vi "Test.vi"(8 "error in (no error)":errorcluster, 10 "board image":T1, 11 "DAQ Board Design in":refnum<class "DAQ Board Design.lvclass">) -> (0 "error out":errorcluster, 2 "pass?":T2, 3 "Test name":string)   [LabVIEW 2018, in "DAQ Board Design.lvclass"]
doc: "Image check for blocks that are common to all types of boards."
uses:
  DAQ Board Design.lvclass
  Common/Pass Fail Boolean.ctl
  Common/Board Image.ctl
  Board Design_class/Board Design.lvclass
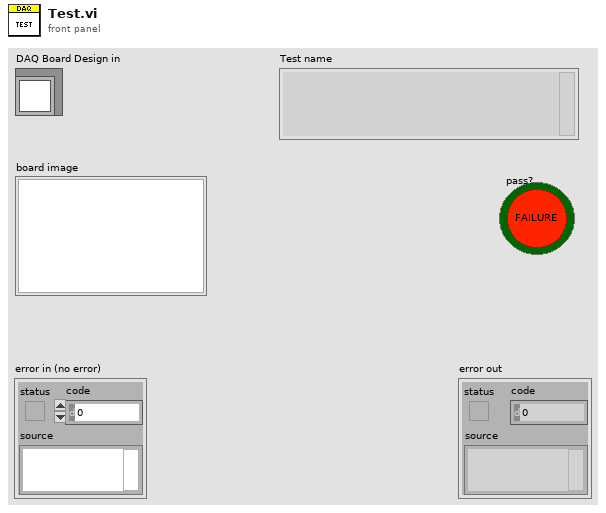
[diagram p1: front panel]
types:
  T1 = typedef "Board Image.ctl" = picture
  T2 = typedef "Pass Fail Boolean.ctl" = bool
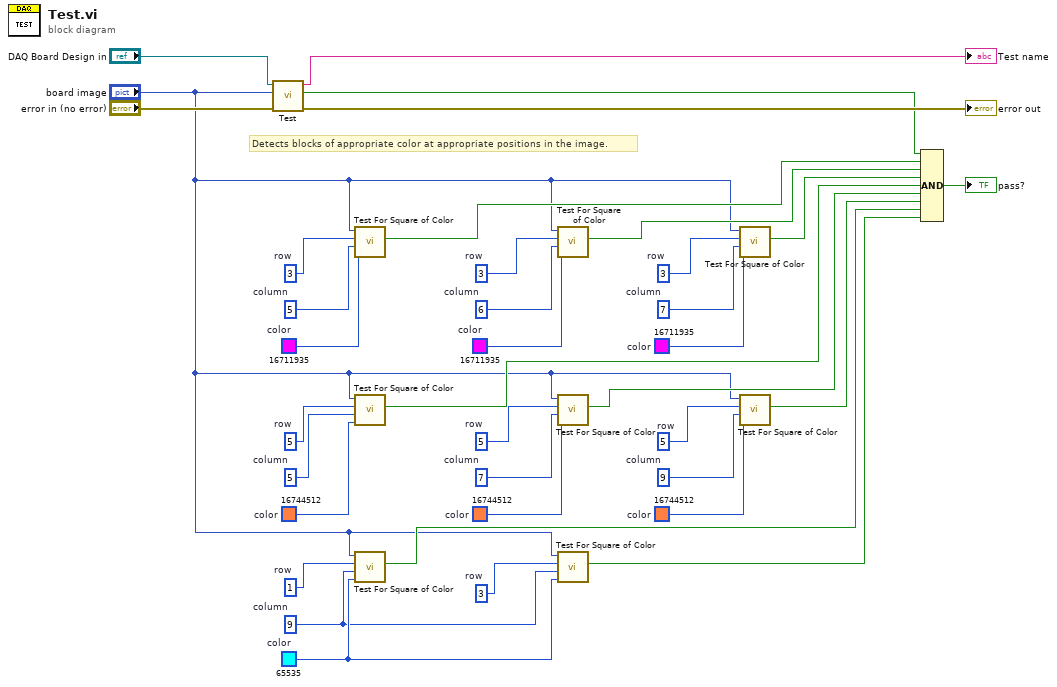
[diagram p0: block diagram]
diagram:
  w5 = u32 65535  # color
  w13 = i16 9  # column
  w12 = i16 5  # row
  w14 = u32 16744512  # color
  w16 = i16 7  # column
  w17 = i16 5  # row
  w15 = u32 16744512  # color
  w19 = i16 5  # column
  w18 = i16 5  # row
  w20 = u32 16744512  # color
  w31 = i16 7  # column
  w32 = i16 3  # row
  w30 = u32 16711935  # color
  w28 = i16 6  # column
  w27 = i16 3  # row
  w29 = u32 16711935  # color
  w25 = i16 5  # column
  w26 = i16 3  # row
  w24 = u32 16711935  # color
  w33 = i16 3  # row
  w4 = i16 9  # column
  w6 = i16 1  # row
  # "Detects blocks of appropriate color at appropriate positions in the image."
  n1 = call-parent "Test.vi"("error in (no error)"="error in (no error)", "board image"="board image", "Board Design in"="DAQ Board Design in") -> ("error out"=→"error out":errorcluster, "pass?"=w2:T2, "Test name"=→"Test name":string)  [unwired: 6 in]
  n2 = call "Test For Square of Color.vi"("color"=w24, "column"=w25, "row"=w26, "board image"="board image") -> ("pass?"=w23:T2)  [unwired: 7 in]
  n3 = call "Test For Square of Color.vi"("color"=w20, "column"=w19, "row"=w18, "board image"="board image") -> ("pass?"=w11:T2)  [unwired: 7 in]
  n4 = call "Test For Square of Color.vi"("color"=w5, "column"=w4, "row"=w6, "board image"="board image") -> ("pass?"=w8:T2)  [unwired: 7 in]
  n5 = call "Test For Square of Color.vi"("color"=w29, "column"=w28, "row"=w27, "board image"="board image") -> ("pass?"=w22:T2)  [unwired: 7 in]
  n6 = call "Test For Square of Color.vi"("color"=w15, "column"=w16, "row"=w17, "board image"="board image") -> ("pass?"=w10:T2)  [unwired: 7 in]
  n7 = call "Test For Square of Color.vi"("color"=w5, "column"=w4, "row"=w33, "board image"="board image") -> ("pass?"=w7:T2)  [unwired: 7 in]
  n8 = call "Test For Square of Color.vi"("color"=w30, "column"=w31, "row"=w32, "board image"="board image") -> ("pass?"=w21:T2)  [unwired: 7 in]
  n9 = call "Test For Square of Color.vi"("color"=w14, "column"=w13, "row"=w12, "board image"="board image") -> ("pass?"=w9:T2)  [unwired: 7 in]
  n10 = Compound Arithmetic op=AND(w2, w23, w22, w21, w11, w10, w9, w8, w7) -> (→"pass?":T2)
